vi "Get JSON Descriptor of Variant.vi"(8 "error in (no error)":errorcluster, 11 "Data Type":variant) -> (0 "error out (no error)":errorcluster, 2 "Total Size":u32, 3 "JSON Descriptor":string)   [LabVIEW 2021, in "DataTypes_CIF_U.lvlib"]
doc: "This helper utility can be used to create as an interface description for a contigous data element (primative, cluster, or 1D array of fixed size). The resulting JSON can be parsed with a standard JSON parser and then the cluster converted using \"Contiguous Structure Converter Assistant.vi\"."
uses:
  DataTypes_CIF_U.lvlib
  Typedef/Errors.ctl
  Typedef/Generic Datatypes.ctl
  SubVIs/DataTypes Error Core.vi
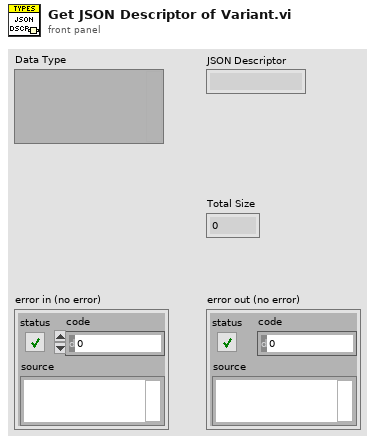
[diagram p1: front panel]
types:
  T1 = typedef "DataTypes_CIF_U.lvlib/Cluster Info.ctl" = cluster{"Name":string[], "Indices":i32[], "Type":T2, "Flat Data Size":u32, "Flat Data Offset":u32, "Memory Size":u32, "Memory Padding":u32, "Memory Offset":u32, "Type Descriptor":i16[]}
  T2 = typedef "NI_Data Type.lvlib/Data Type.ctl" = enum8{"Invalid Type", "Void", "I8", "I16", "I32", "I64", "U8", "U16", "U32", "U64", "Single Float", "Double Float", "Extended Float", "Single Complex", "Double Complex", "Extended Complex", "Enum U8", "Enum U16", "Enum U32", "Enum U64", "Single Float With Unit", "Double Float With Unit", "Extended Float With Unit", "Single Complex with Unit", "Double Complex with Unit", "Extended Complex with Unit", "Boolean", "String", "Path", "Picture", "Tag", "Array", "Cluster", "Variant", "LV Variant", "Waveform", "Timestamp", "Digital Waveform", "Digital Data", "ExpressData", "Refnum", "External Data", "VI", "Poly VI", "LabVIEW Class Instance", "Fixed Point", "Set Collection", "Map Collection"}
  T3 = typedef "DataTypes_CIF_U.lvlib/Errors.ctl" = enum16{"Too few bytes", "Unsupported Type", "Invalid GUID", "Error Parsing JSON"}
  T4 = typedef "DataTypes_CIF_U.lvlib/Generic Datatypes.ctl" = enum16{"Invalid", "Bool", "U8", "I8", "U16", "I16", "U32", "I32", "U64", "I64", "Single Float", "Double Float", "String"}
  T5 = typedef "DataTypes_CIF_U.lvlib/Endian.ctl" = enum16{"Little Endian", "Big Endian"}
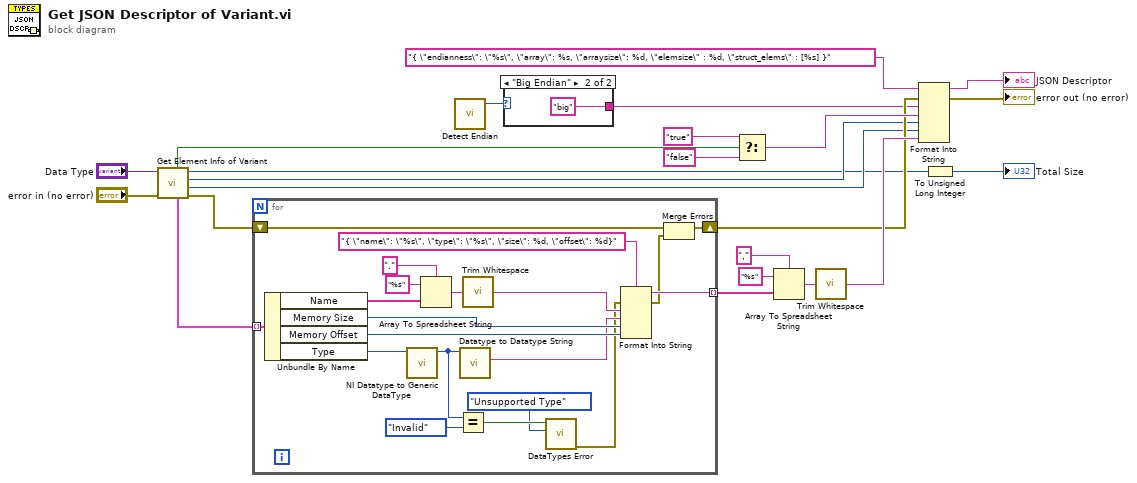
[diagram p0: block diagram]
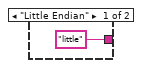
[diagram p2: hidden frame]
diagram:
  n1 = call "Get Element Info of Variant.vi"("error in (no error)"="error in (no error)", "Data Type"="Data Type") -> ("error out"=w5:errorcluster, "Array Element Size"=w4:i32, "Array Size"=w3:i32, "Total Size"=w2:i32, "Cluster Info"=w6:T1[], "Array"=w1:bool)  [unwired: 4 in]
  n2 = for {
    tunnel: w6 -> [w43] mode=indexing
    tunnel: [w36] -> w21 mode=indexing
    shift-right: [w34] -> w13
    shift-left: w5 -> [w32]
    n3 = Unbundle By Name(w43) -> ("Name"=w42:string[], "Memory Size"=w38:u32, "Memory Offset"=w37:u32, "Type"=w30:T2)
    n4 = call "NI Datatype to Generic DataType.vi"("NI Datatype"=w30) -> ("Generic Datatype"=w28:T4)  [unwired: 10 in]
    n5 = Array To Spreadsheet String(delimiter (Tab)=".", array=w42, 3:"%s" ("format string")) -> (spreadsheet string=w40:string)
    n6 = Equal?(x=w28, y=Generic_Datatypes."Invalid") -> (x = y?=w26:bool)
    n7 = call "Datatype to Datatype String.vi"("Generic Datatype"=w28) -> ("Rust String"=w29:string)  [unwired: 9 in, 1 out]
    n8 = call <vilib>:"Trim Whitespace.vi"("string"=w40) -> ("trimmed string"=w39:string)  [unwired: 1 in]
    n9 = call "DataTypes Error.vi"("Error"=Errors."Unsupported Type", "Insert Error"=w26) -> ("error out"=w24:errorcluster)  [unwired: 9 in]
    n10 = Format Into String(format string="{ \"name\": \"%s\", \"type\": \"%s\", \"size\": %d, \"offset\": %d}", error in=w24, w39, w29, w38, w37) -> (resulting string=w36:string, error out=w33:errorcluster)  [unwired: 1 in]
    n11 = Merge Errors(w32, w33) -> (w34:errorcluster)
  }
  n12 = call "Detect Endian.vi"() -> ("Endian"=w10:T5)  [unwired: 5 in]
  n13 = case shown="\"Big Endian\"" w10 {
    tunnel: ["little" "big"] -> w9
    frame "Little Endian" {
    }
    frame "Big Endian" {
    }
  }
  n14 = Select(t="true", s=w1, f="false") -> (s? t:f=w14:string)
  n15 = Array To Spreadsheet String(delimiter (Tab)=",", array=w21, 3:"%s" ("format string")) -> (spreadsheet string=w22:string)
  n16 = call <vilib>:"Trim Whitespace.vi"("string"=w22) -> ("trimmed string"=w19:string)  [unwired: 1 in]
  n17 = Format Into String(format string="{ \"endianness\": \"%s\", \"array\": %s, \"arraysize\": %d, \"elemsize\" : %d, \"struct_elems\" : [%s] }", error in=w13, w9, w14, w3, w4, w19) -> (resulting string=→"JSON Descriptor":string, error out=→"error out (no error)":errorcluster)  [unwired: 1 in]
  n18 = To Unsigned Long Integer(number=w2) -> (unsigned 32bit integer=→"Total Size":u32)
